vi "ModbusTCP_IP.vi"() -> ()   [LabVIEW 2020]
uses:
  <vilib>/Modbus/master/Create Master Instance (TCP).vi
  <vilib>/ErrorRing/Error Ring.xnode
  <vilib>/Modbus/master/Modbus Master.lvclass
panel:
  in  "P1- START - STOP":bool
  in  "P2-Giro Motor":bool
  in  "P3-Velocidad":bool
  out "Horario":bool
  in  "address 2":u16
  in  "starting address":u16
  in  "port (502)":u16=502
  in  "address":string
  out "Velocidad":u16
  out "Vmáx":bool
  out "Vmín":bool
  out "V1":bool
  out "V2":bool
  out "V3":bool
  out "Antihorario":bool
  out "Start Motor":bool
  in  "stop":bool
  # "Alumno: Sánchez Heredia Godo Segundo 1723225287\nCurso: Control de Maquinas Eléctricas\nGrupo Horario: 01L-91G\nCatedrático: Dr. Ing. Temoche Chávez Noe Manuel Jesús"
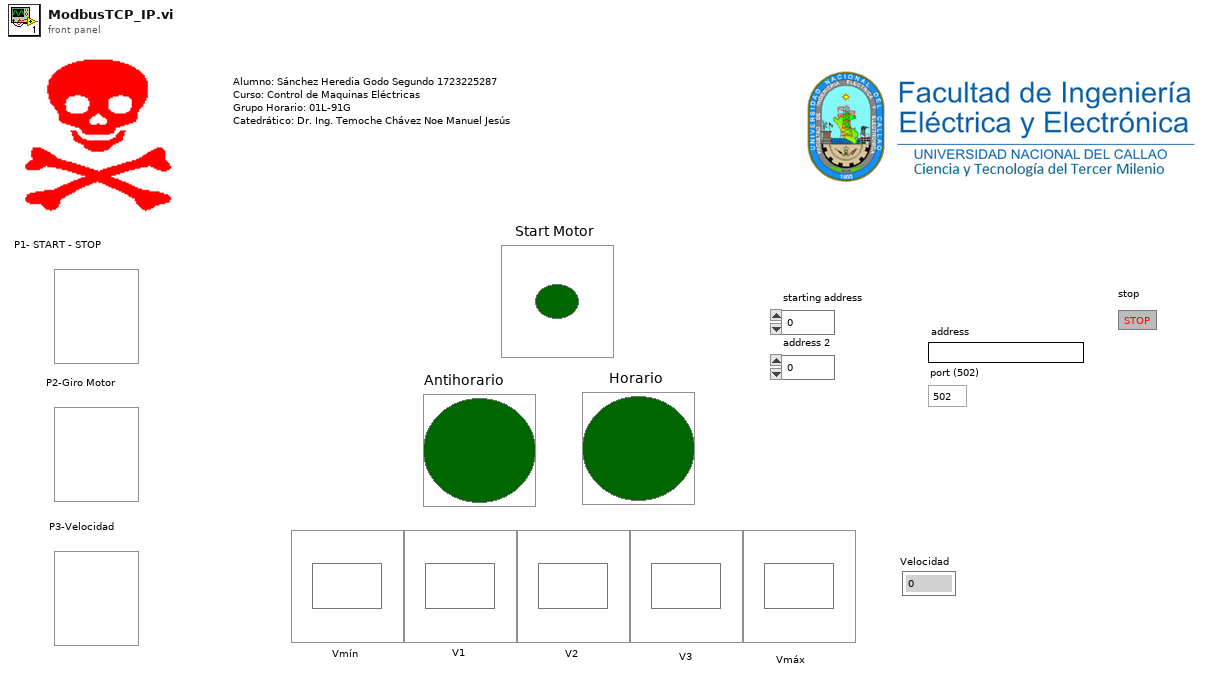
[diagram p1: front panel]
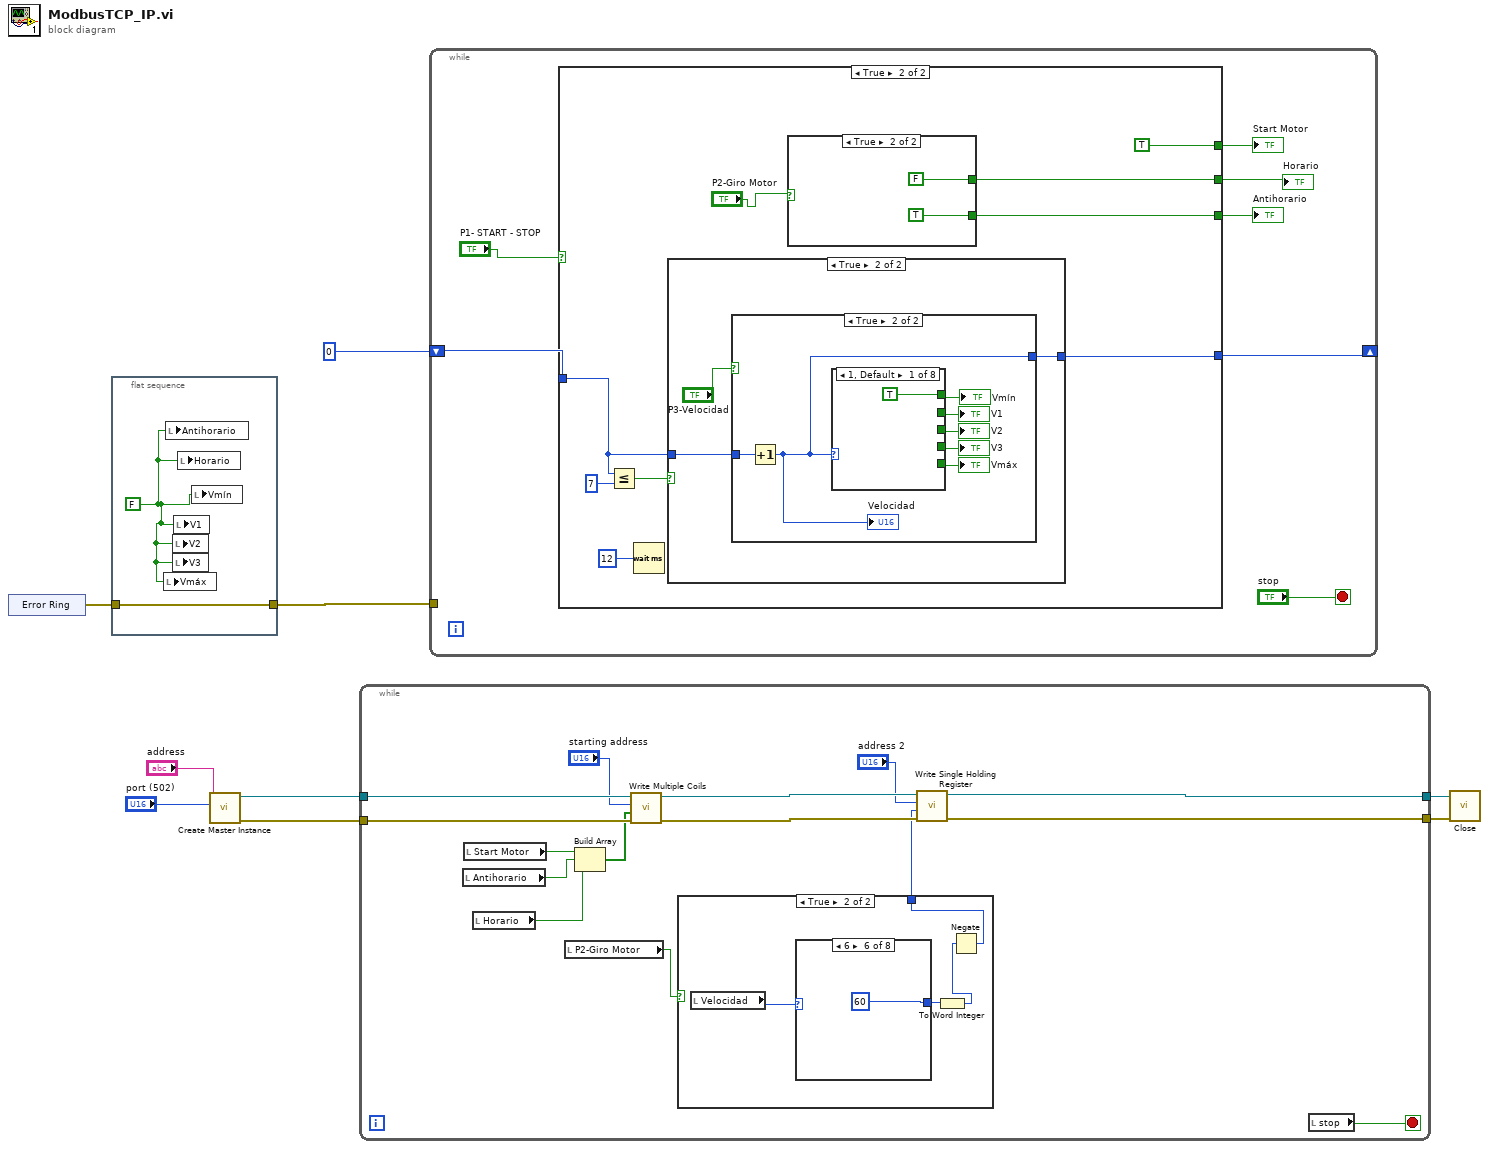
[diagram p0: block diagram]
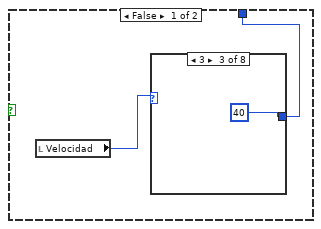
[diagram p2: hidden frame]
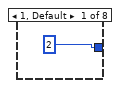
[diagram p3: hidden frame]
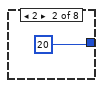
[diagram p4: hidden frame]
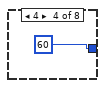
[diagram p5: hidden frame]
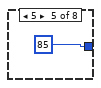
[diagram p6: hidden frame]
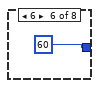
[diagram p7: hidden frame]
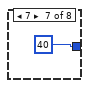
[diagram p8: hidden frame]
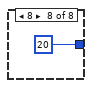
[diagram p9: hidden frame]
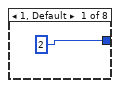
[diagram p10: hidden frame]
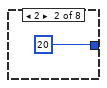
[diagram p11: hidden frame]
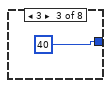
[diagram p12: hidden frame]
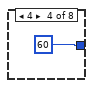
[diagram p13: hidden frame]
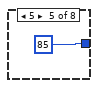
[diagram p14: hidden frame]
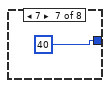
[diagram p15: hidden frame]
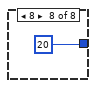
[diagram p16: hidden frame]
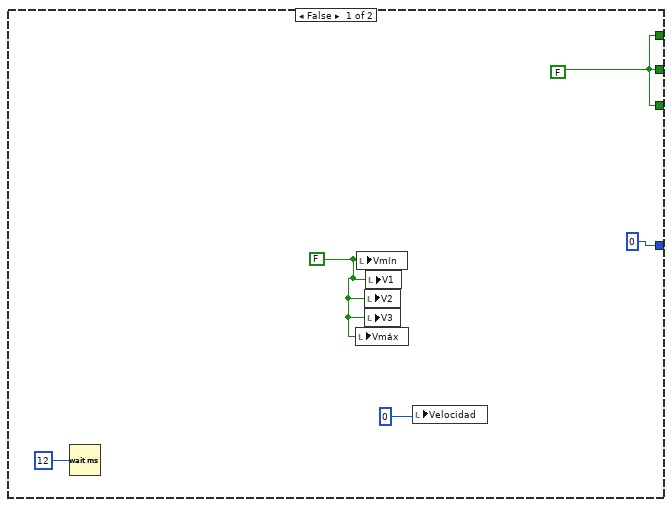
[diagram p17: hidden frame]
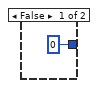
[diagram p18: hidden frame]
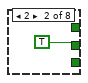
[diagram p20: hidden frame]
diagram:
  n1 = xnode "Error Ring"() -> ("error out"=w7:errorcluster)
  n2 = flat-sequence {
    tunnel: w7 -> [w11]
    tunnel: [w11] -> w8
    frame #0 {
      w10 = FALSE ("Led4")
      n3 = local write "Vmáx"(w10) -> ()
      n4 = local write "Antihorario"(w10) -> ()
      n5 = local write "V2"(w10) -> ()
      n6 = local write "V3"(w10) -> ()
      n7 = local write "V1"(w10) -> ()
      n8 = local write "Horario"(w10) -> ()
      n9 = local write "Vmín"(w10) -> ()
    }
  }
  n10 = call-poly <vilib>:"Create Master Instance.vi"("port (502)"="port (502)", "address"="address") -> ("error out"=w3:errorcluster, "TCP master instance"=w4:refnum<class "Modbus Master.lvclass">)  [unwired: 8 in]
  n11 = while {
    tunnel: w4 -> [w25]
    tunnel: w3 -> [w20]
    tunnel: [w23] -> w2
    tunnel: [w22] -> w1
    stop <- w26 stop-if-true
    n12 = local read "Antihorario"() -> (w14:bool)
    n13 = local read "Start Motor"() -> (w17:bool)
    n14 = local read "Horario"() -> (w16:bool)
    n15 = local read "P2-Giro Motor"() -> (w12:bool)
    n16 = Build Array(w17, w14, w16) -> (w18:bool[])
    n17 = call-dynamic "Write Multiple Coils.vi"("error in (no error)"=w20, "coil values"=w18, "starting address"="starting address", "Modbus master in"=w25) -> ("error out"=w21:errorcluster, "Modbus master out"=w24:refnum<class "Modbus Master.lvclass">)  [unwired: 6 in]
    n18 = case shown="True" w12 {
      tunnel: [w28 w39] -> w13
      frame False {
        n19 = local read "Velocidad"() -> (w27:u16)
        n20 = case shown="3" w27 {
          tunnel: [u16 2 u16 20 u16 40 u16 60 u16 85 u16 60 u16 40 u16 20] -> w28
          frame 1, Default {
          }
          frame 2 {
          }
          frame 3 {
          }
          frame 4 {
          }
          frame 5 {
          }
          frame 6 {
          }
          frame 7 {
          }
          frame 8 {
          }
        }
      }
      frame True {
        n21 = local read "Velocidad"() -> (w40:u16)
        n22 = case shown="6" w40 {
          tunnel: [u16 2 u16 20 u16 40 u16 60 u16 85 u16 60 u16 40 u16 20] -> w38
          frame 1, Default {
          }
          frame 2 {
          }
          frame 3 {
          }
          frame 4 {
          }
          frame 5 {
          }
          frame 6 {
          }
          frame 7 {
          }
          frame 8 {
          }
        }
        n23 = To Word Integer(number=w38) -> (16bit integer=w37:i16)
        n24 = Negate(x=w37) -> (-x=w39:i16)
      }
    }
    n25 = call-dynamic "Write Single Holding Register.vi"("error in (no error)"=w21, "holding register value"=w13, "address"="address 2", "Modbus master in"=w24) -> ("error out"=w22:errorcluster, "Modbus master out"=w23:refnum<class "Modbus Master.lvclass">)  [unwired: 6 in]
    n26 = local read "stop"() -> (w26:bool)
  }
  n27 = while {
    tunnel: w8 -> [_]
    shift-right: [w52] -> _
    shift-left: 0 -> [w51]
    stop <- "stop" stop-if-true
    n28 = case shown="True" "P1- START - STOP" {
      tunnel: [w56 TRUE] -> w55
      tunnel: [w56 w68] -> w50
      tunnel: [w56 w67] -> w54
      tunnel: w51 -> [_ w64]
      tunnel: [0 w63] -> w52
      frame False {
        w59 = FALSE ("Led4")
        w56 = FALSE
        n29 = Wait (ms)(milliseconds to wait=u32 12) -> ()  [unwired: 1 out]
        n30 = local write "Vmáx"(w59) -> ()
        n31 = local write "Vmín"(w59) -> ()
        n32 = local write "V2"(w59) -> ()
        n33 = local write "V3"(w59) -> ()
        n34 = local write "V1"(w59) -> ()
        n35 = local write "Velocidad"(0 ("x+1")) -> ()
      }
      frame True {
        n36 = Less Or Equal?(x=w64, y=7) -> (x <= y?=w65:bool)
        n37 = Wait (ms)(milliseconds to wait=u32 12) -> ()  [unwired: 1 out]
        n38 = case shown="True" w65 {
          tunnel: [0 w73] -> w63
          tunnel: w64 -> [_ w72]
          frame False {
          }
          frame True {
            n39 = case shown="True" "P3-Velocidad" {
              tunnel: [w74 w81] -> w73
              tunnel: w72 -> [w74 w75]
              frame False {
              }
              frame True {
                n40 = Increment(x=w75) -> (x+1=w81:i32)
                "Velocidad" <- w81
                n41 = case shown="1, Default" w81 {
                  tunnel: [TRUE _ _ _ _ _ _ _] -> w80
                  tunnel: [_ TRUE _ _ _ _ _ TRUE] -> w79
                  tunnel: [_ _ _ TRUE _ TRUE _ _] -> w77
                  tunnel: [_ _ _ _ TRUE _ _ _] -> w76
                  tunnel: [_ _ TRUE _ _ _ TRUE _] -> w78
                  frame 1, Default {
                  }
                  frame 2 {
                  }
                  frame 3 {
                  }
                  frame 4 {
                  }
                  frame 5 {
                  }
                  frame 6 {
                  }
                  frame 7 {
                  }
                  frame 8 {
                  }
                }
                "Vmáx" <- w76
                "Vmín" <- w80
                "V1" <- w79
                "V2" <- w78
                "V3" <- w77
              }
            }
          }
        }
        n42 = case shown="True" "P2-Giro Motor" {
          tunnel: [TRUE FALSE] -> w68
          tunnel: [FALSE TRUE] -> w67
          frame False {
          }
          frame True {
          }
        }
      }
    }
    "Start Motor" <- w55
    "Antihorario" <- w54
    "Horario" <- w50
  }
  n43 = call-dynamic "Close.vi"("error in (no error)"=w1, "Modbus master in"=w2) -> ()  [unwired: 9 in, 1 out]
